vi "Press Button.vi"(0 "GEA2 Reference In":refnum<k24>, 7 "Button":T1=enum."SW201 - My Cycle", 11 "Error In":errorcluster) -> (4 "GEA2 Reference Out":refnum<k24>, 15 "Error Out":errorcluster)   [LabVIEW 2018, in "TLMB.lvlib"]
doc: "This VI is used to perform button presses on the HEUI and LEUI."
uses:
  Projects/TLMB.lvlib
  type defs/UI Buttons.ctl
  D:/Common/LabVIEW GEA2 Toolkit/source/GEA3 DLL Source/GeaCommunication.dll
  Common/LabVIEW GEA2 Toolkit/source/GEA3 DLL Source/GeaCommunication.dll
  Common/LabVIEW GEA2 Toolkit/GEA3/type defs/ERD Write Data In.ctl
  Common/LabVIEW GEA2 Toolkit/GEA3/type defs/Data Type.ctl
  Common/LabVIEW GEA2 Toolkit/GEA3/type defs/Source_Destination.ctl
  C:/Users/iallatyp/Desktop/New folder/GEA3/library/GEA2_Toolkit.lvlib
panel:
  in  "Standalone?":bool
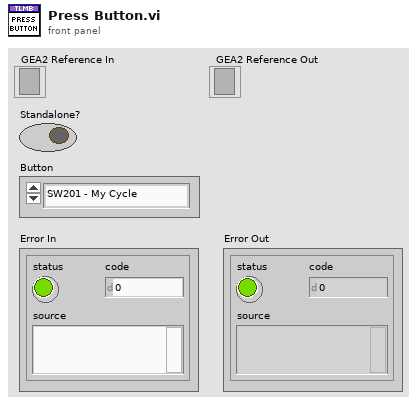
[diagram p1: front panel]
types:
  T1 = typedef "TLMB.lvlib/UI Buttons.ctl" = enum16{"Switch Off", "SW201 - My Cycle", "SW202 - Delay Wash", "SW203 - Extra Rinse", "SW204 - Signal / Volume", "SW205 - Spin", "SW206 - Deep Rinse / Fab Soft", "SW207 - Soil", "SW208 - Auto Soak", "SW209 - Temp", "SW210 - Warm Rinse", "SW211 - Deep Fill", "SW212 - Stain Remover", "SW213 - Power", "SW222 - Control Lock", "SW214 - Start / Pause", "SW301 - Start/Pause LE", "SW302 - Option Button LE", "SW201/212 - Bulk Flush"}
  T2 = typedef "GEA2_Toolkit.lvlib/ERD Write Data In.ctl" = cluster{"ERD Number":u16, "Data Type":T3, "Data":string}
  T3 = typedef "GEA2_Toolkit.lvlib/Data Type.ctl" = enum16{"string", "boolean", "uint8_t", "uint16_t", "uint32_t", "uint64_t", "int8_t", "int16_t", "int32_t", "int64_t"}
  T4 = typedef "GEA2_Toolkit.lvlib/Source_Destination.ctl" = cluster{"Source":u8, "Destination":u8}
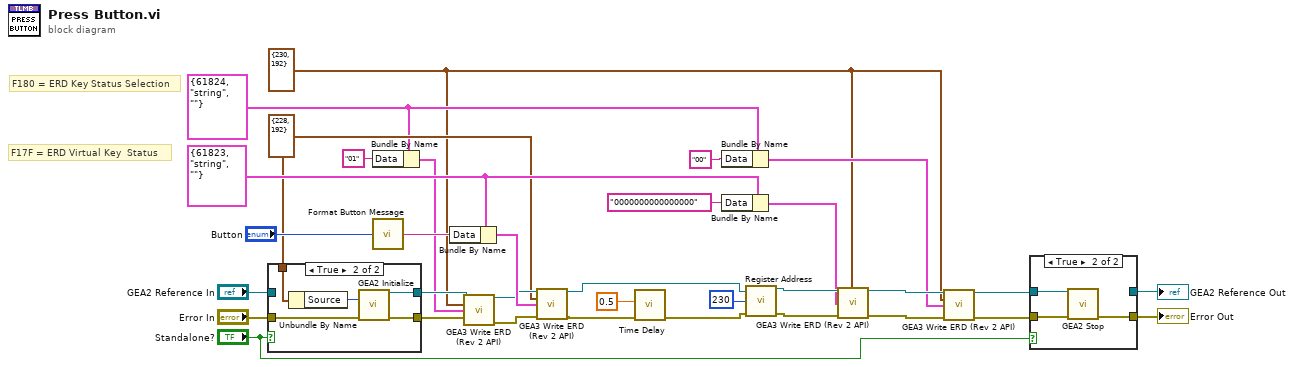
[diagram p0: block diagram]
diagram:
  w4 = T2 {"ERD Number"=61824, "Data Type"=enum."string", "Data"=""} ("ERD Write Data In")
  w1 = T4 {"Source"=230, "Destination"=192} ("GEA Inputs")
  w11 = T4 {"Source"=228, "Destination"=192} ("GEA Inputs")
  w24 = T2 {"ERD Number"=61823, "Data Type"=enum."string", "Data"=""} ("ERD Write Data In")
  # "F17F = ERD Virtual Key  Status"
  # "F180 = ERD Key Status Selection"
  n1 = case shown="True" "Standalone?" {
    tunnel: "Error In" -> [w34 w40]
    tunnel: [w34 w39] -> w15
    tunnel: "GEA2 Reference In" -> [w35 _]
    tunnel: [w35 w38] -> w13
    tunnel: w11 -> [_ w36]
    frame False {
    }
    frame True {
      n2 = Unbundle By Name(w36) -> ("Source"=w37:u8)
      n3 = call "GEA2 Initialize.vi"("Source Address"=w37, "error in"=w40) -> ("GEA2 Reference Out"=w38:refnum<k24>, "error out"=w39:errorcluster)  [unwired: 11 in, 1 out]
    }
  }
  n4 = Bundle By Name(cluster=w4, "Data"="01") -> (w10:T2)
  n5 = call "Format Button Message.vi"("Switch"="Button") -> ("Switch Message"=w26:string)  [unwired: 14 in]
  n6 = Bundle By Name(cluster=w24, "Data"=w26) -> (w21:T2)
  n7 = call "GEA3 Write ERD (Rev 2 API).vi"("GEA2 Reference In"=w13, "GEA Inputs"=w1, "ERD Write Data In"=w10, "Error In"=w15) -> ("GEA2 Reference Out"=w12:refnum<k24>, "Error Out"=w14:errorcluster)  [unwired: 9 in, 1 out]
  n8 = call "GEA3 Write ERD (Rev 2 API).vi"("GEA2 Reference In"=w12, "GEA Inputs"=w11, "ERD Write Data In"=w21, "Error In"=w14) -> ("GEA2 Reference Out"=w19:refnum<k24>, "Error Out"=w20:errorcluster)  [unwired: 9 in, 1 out]
  n9 = call "Time Delay"("error in (no error)"=w20, "Delay Time (s)"=0.5) -> ("error out"=w22:errorcluster)  [unwired: 9 in]
  n10 = Bundle By Name(cluster=w4, "Data"="00") -> (w2:T2)
  n11 = Bundle By Name(cluster=w24, "Data"="0000000000000000" ("Message")) -> (w16:T2)
  n12 = call "Register Address.vi"("GEA2 Reference In"=w19, "Address"=u8 230 ("Source"), "Error In"=w22) -> ("GEA2 Reference Out"=w18:refnum<k24>, "Error Out"=w17:errorcluster)  [unwired: 11 in]
  n13 = call "GEA3 Write ERD (Rev 2 API).vi"("GEA2 Reference In"=w18, "GEA Inputs"=w1, "ERD Write Data In"=w16, "Error In"=w17) -> ("GEA2 Reference Out"=w8:refnum<k24>, "Error Out"=w7:errorcluster)  [unwired: 9 in, 1 out]
  n14 = call "GEA3 Write ERD (Rev 2 API).vi"("GEA2 Reference In"=w8, "GEA Inputs"=w1, "ERD Write Data In"=w2, "Error In"=w7) -> ("GEA2 Reference Out"=w5:refnum<k24>, "Error Out"=w6:errorcluster)  [unwired: 9 in, 1 out]
  n15 = case shown="True" "Standalone?" {
    tunnel: [w41 w45] -> w29
    tunnel: w5 -> [w42 w44]
    tunnel: [w42 _] -> w28
    tunnel: w6 -> [w41 w43]
    frame False {
    }
    frame True {
      n16 = call "GEA2 Stop.vi"("GEA2 Reference In"=w44, "Error In"=w43) -> ("Error Out"=w45:errorcluster)  [unwired: 13 in]
    }
  }
  "Error Out" <- w29
  "GEA2 Reference Out" <- w28
